vi "move Scanner.vi"(5 "Axis":u16(ring) items=["X-Axis", "Y-Axis"], 6 "error in (no error)":errorcluster, 7 "Position":dbl(slide)=-0.10452961921691895 scale=-6.0..6.0, 8 "GalvoControl":refnum<class "Probe.lvclass">, 9 "OCTDevice":refnum<class "OCT Device.lvclass">) -> (0 "error out":errorcluster, 2 "GalvoControl":refnum<class "Probe.lvclass">, 3 "OCTDevice":refnum<class "OCT Device.lvclass">)   [LabVIEW 2018]
doc: "Moves the given galvo scanner to a position in mm relative to the galvo's home position. Device and GaloControl/Probe instances need to be initialized before using this VI."
uses:
  SpectralRadar/LabVIEW/2012/user.lib/SpectralRadar.llb/OCT Device.lvclass
  SpectralRadar/LabVIEW/2012/user.lib/SpectralRadar.llb/Probe.lvclass
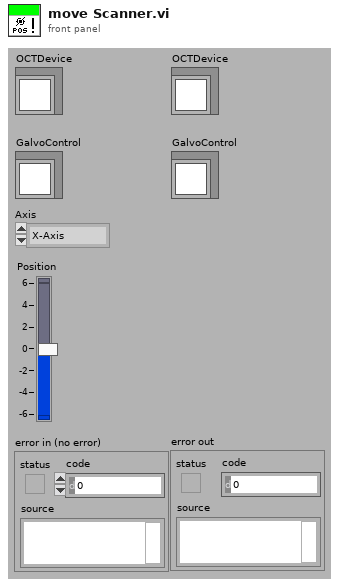
[diagram p1: front panel]
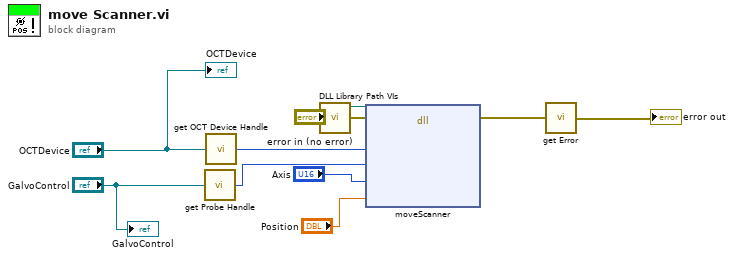
[diagram p0: block diagram]
diagram:
  n1 = call "get Probe Handle.vi"("GalvoControl"="GalvoControl") -> ("Galvo Control Handle"=w6:u64)
  n2 = call "get OCT Device Handle.vi"("OCTDevice"="OCTDevice") -> ("OCT Device Handle"=w9:u64)
  n3 = call "DLL Library Path VIs.vi"() -> ("SpectralRadarDLL"=w1:path)  [unwired: 8 in, 3 out]
  n4 = dll-call lib="C:/Project/SerialSectOCT - FFT GPU/SerialSectOCT/Labview Software/DLL/SpectralRadar.dll" fn="moveScanner"(path in=w1, error in="error in (no error)", "OCT Device Handle"=w9, "Probe Handle"=w6, "Axis"="Axis", "Position"="Position") -> (error out=w3:errorcluster)  [unwired: 6 in, 1 out]
  n5 = call "get Error.vi"("error in (no error)"=w3) -> ("error out"=→"error out":errorcluster)
  "OCTDevice" <- "OCTDevice"
  "GalvoControl" <- "GalvoControl"
